vi "Disconnect All.vi"(8 "error in (no error)":errorcluster, 11 "NI-SWITCH Consumer in":refnum<class "%DEVICE% Consumer.lvclass">) -> (0 "error out":errorcluster, 3 "NI-SWITCH Consumer out":refnum<class "%DEVICE% Consumer.lvclass">)   [LabVIEW 2017, in "%DEVICE% Messaging.lvlib" / "%DEVICE% Consumer.lvclass"]
uses:
  %DEVICE% Consumer.lvclass
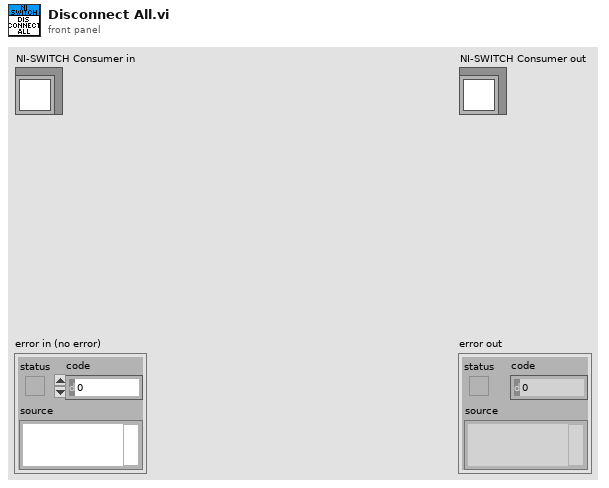
[diagram p1: front panel]
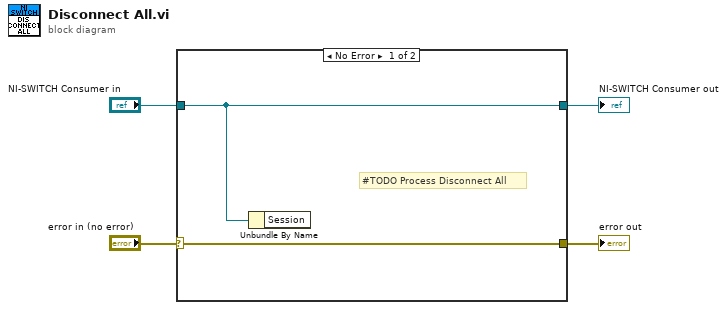
[diagram p0: block diagram]
diagram:
  n1 = case shown="No Error" "error in (no error)" {
    selector: "error in (no error)" -> [w5 w8]
    tunnel: [w5 w8] -> w3
    tunnel: [w6 w7] -> w1
    tunnel: "NI-SWITCH Consumer in" -> [w6 w7]
    frame No Error {
      # "#TODO Process Disconnect All"
      n2 = Unbundle By Name(w6) -> ()  [unwired: 1 out]
    }
    frame Error {
    }
  }
  "error out" <- w3
  "NI-SWITCH Consumer out" <- w1
